vi "GetImageData.vi"(7 "error in (no error)":errorcluster, 10 "Image":T1) -> (0 "error out":errorcluster, 3 "Array":dbl[](array[numeric]))   [LabVIEW 2016]
uses:
  <vilib>/vision/Image Controls.llb/IMAQ Image.ctl
  <vilib>/Analysis/baseanly.llb/Mean (DBL).vi
  <vilib>/Analysis/NI_AALBase.lvlib
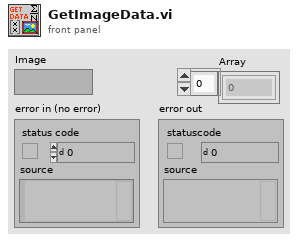
[diagram p1: front panel]
types:
  T1 = typedef "IMAQ Image.ctl" = refnum<image>
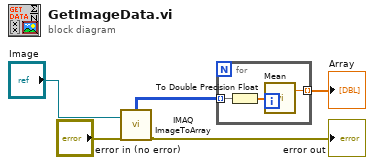
[diagram p0: block diagram]
diagram:
  n1 = call "IMAQ ImageToArray"("error in (no error)"="error in (no error)", "Image"="Image") -> ("error out"=→"error out":errorcluster, "Image Pixels (U8)"=w4:u8[][])  [unwired: 2 in, 3 out]
  n2 = for {
    tunnel: [w8] -> w5 mode=indexing
    tunnel: w4 -> [w7] mode=indexing
    n3 = To Double Precision Float(number=w7) -> (double precision float=w6:dbl[])
    n4 = call-poly <vilib>:"Mean.vi"("X"=w6) -> ("mean"=w8:dbl)  [unwired: 1 out]
  }
  "Array" <- w5
